vi "Scan Engine.vi"() -> ()   [LabVIEW 2018]
uses:
  Controls/QueueNames.ctl
  Controls/Queue Manager Actions.ctl
  Controls/MessagePacket.ctl
panel:
  in  "Error In":errorcluster
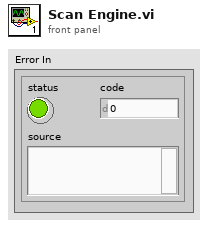
[diagram p1: front panel]
types:
  T1 = typedef "MessagePacket.ctl" = cluster{"Message":string, "Parameter":variant}
  T2 = typedef "Queue Manager Actions.ctl" = enum16{"Init", "Enqueue", "Enqueue All", "Preview Queue", "Dequeue", "Get Status", "Flush Queue", "Flush All Queues", "Release All Queues", "Release Queue", "Enqueue at Opposite End"}
  T3 = typedef "QueueNames.ctl" = enum16{"Main GUI", "Main Scan Processor", "Main Processing", "Main Saving", "Main Display", "Main Table Stage GUI", "Main Table Stage Proc.", "Scan Engine", "Vibratome GUI", "Vibratome Processor", "Slice Engine"}
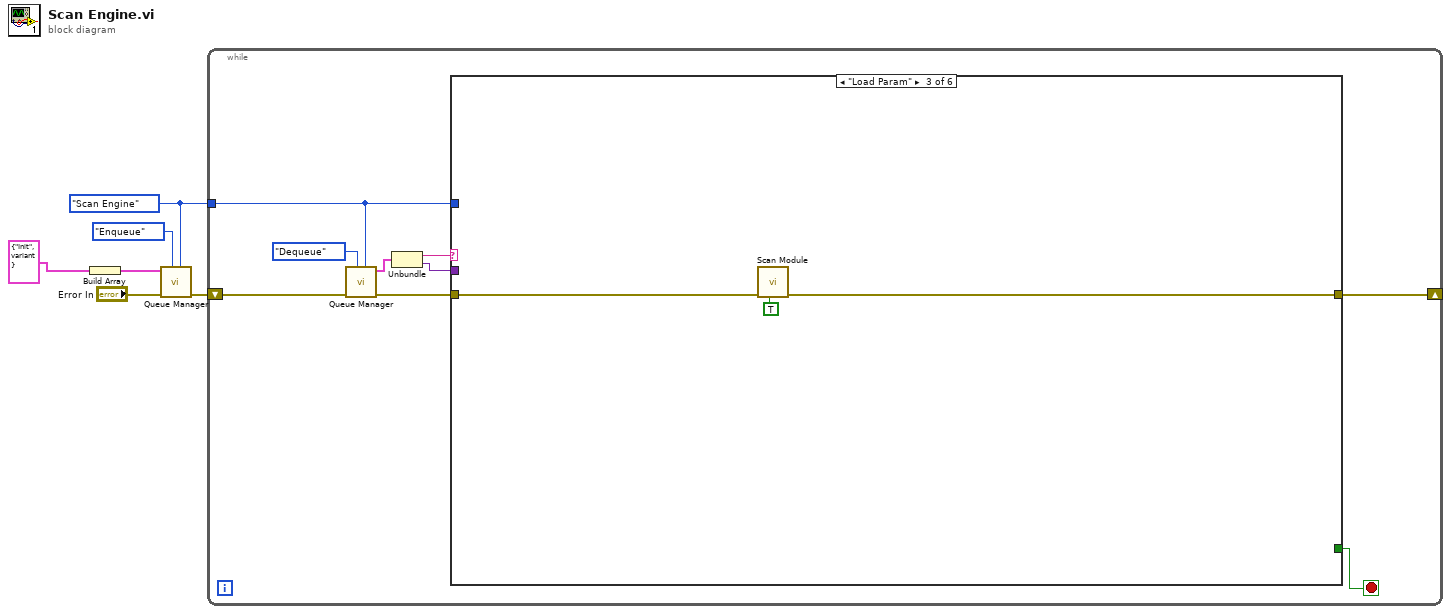
[diagram p0: block diagram]
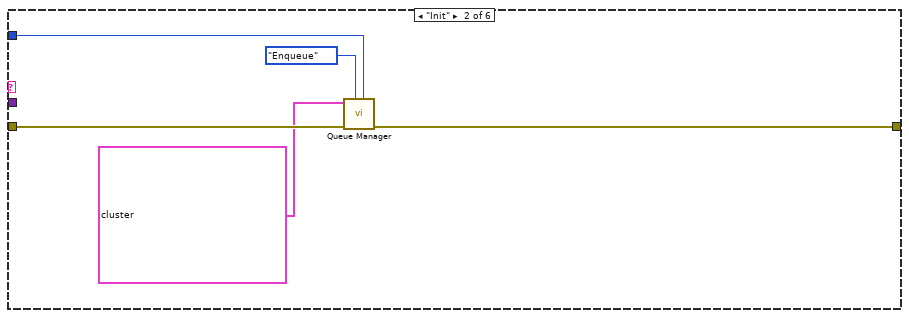
[diagram p3: hidden frame]
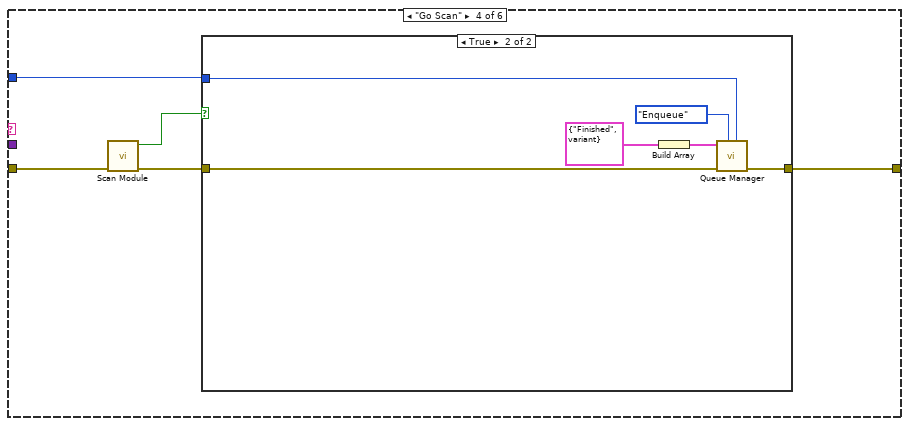
[diagram p4: hidden frame]
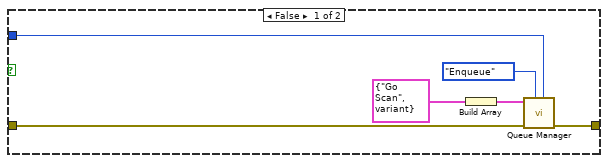
[diagram p5: hidden frame]
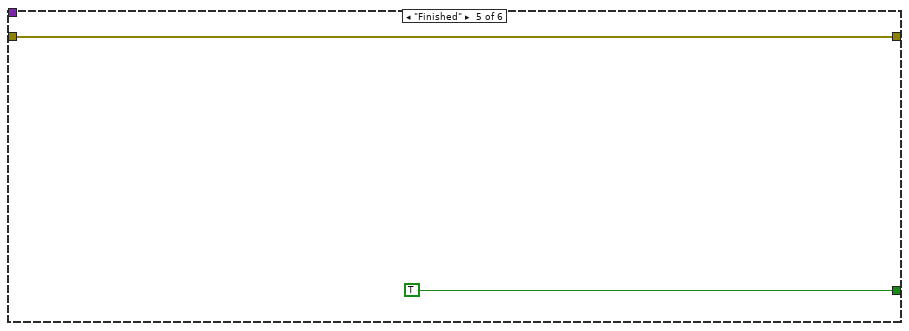
[diagram p6: hidden frame]
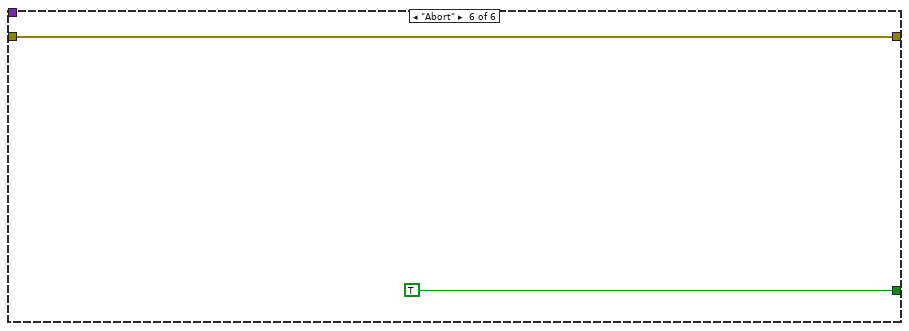
[diagram p7: hidden frame]
diagram:
  w1 = QueueNames."Scan Engine" ("Queue Name")
  n1 = Build Array(T1 {"Message"="Init", "Parameter"=variant} ("Message Packet")) -> (w2:T1[])
  n2 = call "Queue Manager.vi"("Queue Name"=w1, "Action"=Queue_Manager_Actions."Enqueue", "Error In"="Error In", "Message Packet Array"=w2) -> ("Error Out"=w4:errorcluster)  [unwired: 3 in, 4 out]
  n3 = while {
    tunnel: w1 -> [w7]
    shift-right: [w8] -> _
    shift-left: w4 -> [w15]
    stop <- w12 stop-if-true
    n4 = call "Queue Manager.vi"("Queue Name"=w7, "Action"=Queue_Manager_Actions."Dequeue", "Error In"=w15) -> ("Error Out"=w9:errorcluster, "Message Packet [Out]"=w13:T1)  [unwired: 4 in, 3 out]
    n5 = Unbundle(w13) -> ("Message"=w11:string, "Parameter"=w10:variant)
    n6 = case shown="\"Load Param\"" w11 {
      tunnel: [_ _ _ _ TRUE TRUE] -> w12
      tunnel: w10 -> [_ _ _ _ _ _]
      tunnel: w9 -> [w16 w21 w24 w29 w42 w44]
      tunnel: [w16 w20 w23 w27 w42 w44] -> w8
      tunnel: w7 -> [_ w19 _ w26 _ _]
      frame "Error", Default {
      }
      frame "Init" {
        n7 = call "Queue Manager.vi"("Queue Name"=w19, "Action"=Queue_Manager_Actions."Enqueue", "Error In"=w21, "Message Packet Array"=T1[] [{"Message"="Load Param", "Parameter"=variant}, {"Message"="Go Scan", "Parameter"=variant}]) -> ("Error Out"=w20:errorcluster)  [unwired: 3 in, 4 out]
      }
      frame "Load Param" {
        n8 = call "Scan Module.vi"("Init"=TRUE, "Error In"=w24) -> ("Error Out"=w23:errorcluster)  [unwired: 6 in, 3 out]
      }
      frame "Go Scan" {
        n9 = call "Scan Module.vi"("Error In"=w29) -> ("Error Out"=w25:errorcluster, "Finished?"=w28:bool)  [unwired: 7 in, 2 out]
        n10 = case shown="True" w28 {
          tunnel: w25 -> [w35 w41]
          tunnel: [w34 w40] -> w27
          tunnel: w26 -> [w33 w39]
          frame False {
            n11 = Build Array(T1 {"Message"="Go Scan", "Parameter"=variant} ("Message Packet")) -> (w30:T1[])
            n12 = call "Queue Manager.vi"("Queue Name"=w33, "Action"=Queue_Manager_Actions."Enqueue", "Error In"=w35, "Message Packet Array"=w30) -> ("Error Out"=w34:errorcluster)  [unwired: 3 in, 4 out]
          }
          frame True {
            n13 = Build Array(T1 {"Message"="Finished", "Parameter"=variant} ("Message Packet")) -> (w36:T1[])
            n14 = call "Queue Manager.vi"("Queue Name"=w39, "Action"=Queue_Manager_Actions."Enqueue", "Error In"=w41, "Message Packet Array"=w36) -> ("Error Out"=w40:errorcluster)  [unwired: 3 in, 4 out]
          }
        }
      }
      frame "Finished" {
      }
      frame "Abort" {
      }
    }
  }
